vi "Burst.vi"(0 "RFFE Command in":refnum<class "RFFE Command.lvclass">, 1 "Bus Number":i32, 5 "instrument handle in":refnum<k15>, 11 "error in (no error)":errorcluster) -> (4 "RFFE Command out":refnum<class "RFFE Command.lvclass">, 6 "instrument handle out":refnum<k15>, 15 "error out":errorcluster)   [LabVIEW 2018, in "MIPI RFFE API.lvlib" / "RFFE Command.lvclass"]
uses:
  RFFE Command.lvclass
  <instrlib>/niDigital/niDigital.llb/niDigital Burst Pattern (Burst Only).vi
  MIPI RFFE API.lvlib
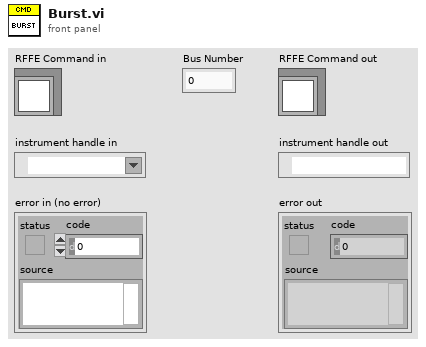
[diagram p1: front panel]
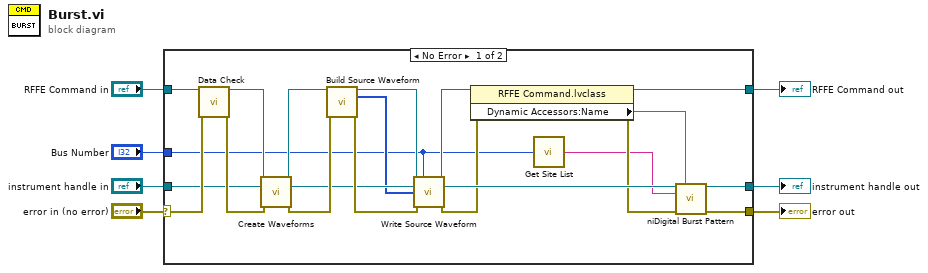
[diagram p0: block diagram]
diagram:
  n1 = case shown="No Error" "error in (no error)" {
    selector: "error in (no error)" -> [w23 w31]
    tunnel: [w20 w31] -> w6
    tunnel: [w21 w30] -> w4
    tunnel: "RFFE Command in" -> [w27 w30]
    tunnel: "instrument handle in" -> [w22 w29]
    tunnel: [w18 w29] -> w2
    tunnel: "Bus Number" -> [w9 _]
    frame No Error {
      n2 = call-dynamic "Data Check.vi"("RFFE Command in"=w27, "error in (no error)"=w23) -> ("RFFE Command out"=w28:refnum<class "RFFE Command.lvclass">, "error out"=w25:errorcluster)  [unwired: 12 in]
      n3 = call-dynamic "Create Waveforms.vi"("RFFE Command in"=w28, "instrument handle in"=w22, "error in (no error)"=w25) -> ("RFFE Command out"=w26:refnum<class "RFFE Command.lvclass">, "instrument handle out"=w14:refnum<k15>, "error out"=w24:errorcluster)  [unwired: 10 in]
      n4 = call-dynamic "Build Source Waveform.vi"("RFFE Command in"=w26, "error in (no error)"=w24) -> ("RFFE Command out"=w17:refnum<class "RFFE Command.lvclass">, "Source Waveform"=w12:u32[], "error out"=w15:errorcluster)  [unwired: 11 in]
      n5 = call-dynamic "Write Source Waveform.vi"("RFFE Command in"=w17, "Bus Number"=w9, "instrument handle"=w14, "Waveform Data"=w12, "error in (no error)"=w15) -> ("RFFE Command out"=w16:refnum<class "RFFE Command.lvclass">, "instrument handle out"=w13:refnum<k15>, "error out"=w11:errorcluster)  [unwired: 8 in]
      n6 = property class="RFFE Command.lvclass"(reference=w16, error in=w11) -> (reference out=w21:refnum<class "RFFE Command.lvclass">, error out=w10:errorcluster, "Dynamic Accessors:Name"=w19:string)
      n7 = call "Get Site List.vi"("Bus Number"=w9) -> ("Site List"=w8:string)  [unwired: 14 in]
      n8 = call-poly <instrlib>:"niDigital Burst Pattern.vi"("instrument handle"=w13, "start label"=w19, "site list"=w8, "error in"=w10) -> ("instrument handle out"=w18:refnum<k15>, "error out"=w20:errorcluster)  [unwired: 10 in]
    }
    frame Error {
    }
  }
  "error out" <- w6
  "RFFE Command out" <- w4
  "instrument handle out" <- w2
